vi "#253_MAV_MSG_STATUSTEXT_DECODE.vi"(11 "mavlink_payload":u8[](array[numeric])) -> (3 "STATUSTEXT":T1(array[cluster]))   [LabVIEW 2023]
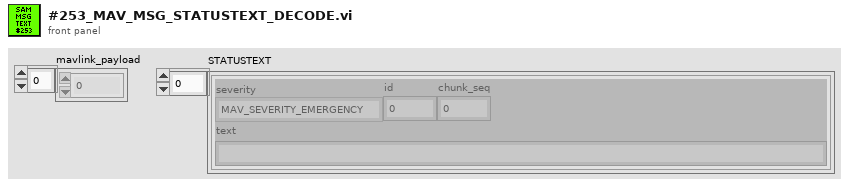
[diagram p1: front panel]
types:
  T1 = cluster{"severity":enum8{"MAV_SEVERITY_EMERGENCY", "MAV_SEVERITY_ALERT", "MAV_SEVERITY_CRITICAL", "MAV_SEVERITY_ERROR", "MAV_SEVERITY_WARNING", "MAV_SEVERITY_NOTICE", "MAV_SEVERITY_INFO", "MAV_SEVERITY_DEBUG"}, "id":u16, "chunk_seq":u8, "text":string}[]
  T2 = enum8{"MAV_SEVERITY_EMERGENCY", "MAV_SEVERITY_ALERT", "MAV_SEVERITY_CRITICAL", "MAV_SEVERITY_ERROR", "MAV_SEVERITY_WARNING", "MAV_SEVERITY_NOTICE", "MAV_SEVERITY_INFO", "MAV_SEVERITY_DEBUG"}
  T3 = cluster{"severity":enum8{"MAV_SEVERITY_EMERGENCY", "MAV_SEVERITY_ALERT", "MAV_SEVERITY_CRITICAL", "MAV_SEVERITY_ERROR", "MAV_SEVERITY_WARNING", "MAV_SEVERITY_NOTICE", "MAV_SEVERITY_INFO", "MAV_SEVERITY_DEBUG"}, "id":u16, "chunk_seq":u8, "text":string}
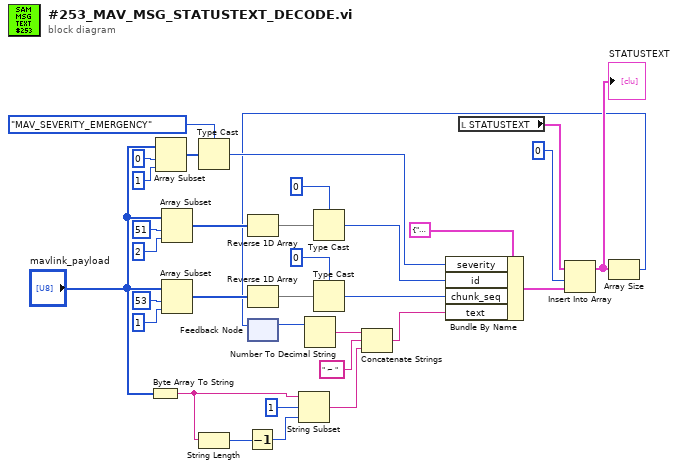
[diagram p0: block diagram]
diagram:
  n1 = Byte Array To String(unsigned byte array="mavlink_payload") -> (string=w30:string)
  n2 = Array Subset(array="mavlink_payload", index=0 ("Index"), length=1) -> (w24:u8[])
  n3 = Array Subset(array="mavlink_payload", index=51 ("Index"), length=2) -> (w19:u8[])
  n4 = Array Subset(array="mavlink_payload", index=53 ("Index"), length=1) -> (w13:u8[])
  n5 = Type Cast(type=T2."MAV_SEVERITY_EMERGENCY" ("severity"), x=w24) -> (*(type *) &x=w23:T2)
  n6 = String Length(string=w30) -> (length=w31:i32)
  n7 = Decrement(x=w31) -> (x-1=w32:i32)
  n8 = Reverse 1D Array(array=w19) -> (reversed array=w18:u8[])
  n9 = Reverse 1D Array(array=w13) -> (reversed array=w12:u8[])
  n10 = feedback #1() -> (w2:i32)  [unwired: 1 in]
  n11 = String Subset(string=w30, offset (0)=1, length (rest)=w32) -> (substring=w28:string)
  n12 = Number To Decimal String(number=w2) -> (decimal integer string=w3:string)  [unwired: 1 in]
  n13 = Type Cast(type=u16 0 ("Index"), x=w18) -> (*(type *) &x=w16:u16)
  n14 = Type Cast(type=u8 0 ("Index"), x=w12) -> (*(type *) &x=w10:u8)
  n15 = Concatenate Strings(w3, " ~ " ("string"), w28) -> (w27:string)
  n16 = Bundle By Name(cluster=T3 {"severity"=enum."MAV_SEVERITY_EMERGENCY", "id"=0, "chunk_seq"=0, "text"=""} ("STATUSTEXT"), "severity"=w23, "id"=w16, "chunk_seq"=w10, "text"=w27) -> (w9:T3)
  n17 = local read "STATUSTEXT"() -> (w5:T1)
  n18 = Insert Into Array(array=w5, index=0, new element=w9) -> (w4:T1)
  "STATUSTEXT" <- w4
  n19 = Array Size(array=w4) -> (size(s)=w1:i32)
  n20 = feedback-in #1(w1) -> ()
